vi "conect and open B.vi"(4 "Slot":u32, 5 "Bus":u32, 6 "Remote Machine":string="192.168.1.218", 7 "Card ID":string) -> (0 "error out":errorcluster {"code" format="%.0x"}, 2 "find?":bool, 3 "Output Handle":cluster{"Session":u32, "Card number":u32})   [LabVIEW 2018]
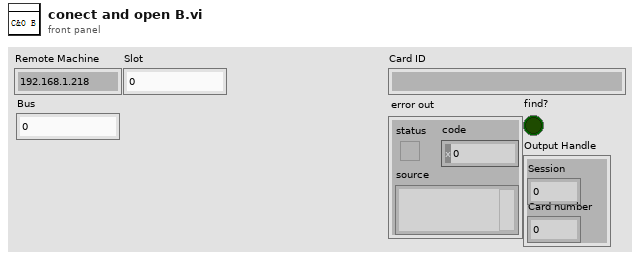
[diagram p1: front panel]
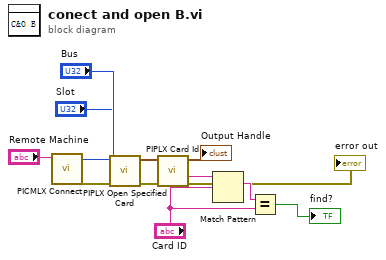
[diagram p0: block diagram]
diagram:
  n1 = call <instrlib>:"PICMLX Connect.vi"("Remote Machine"="Remote Machine") -> ("error out"=w12:errorcluster, "Session"=w13:u32)  [unwired: 8 in]
  n2 = call <instrlib>:"PIPLX Open Specified Card.vi"("error in"=w12, "Slot"="Slot", "Bus"="Bus", "Session"=w13) -> ("error out"=w11:errorcluster, "Output Handle"=w10:cluster{"Session":u32, "Card number":u32})  [unwired: 6 in]
  n3 = call <instrlib>:"PIPLX Card Id.vi"("error in"=w11, "Input Handle"=w10) -> ("error out"=→"error out":errorcluster, "Card ID"=w9:string, "Output Handle"=→"Output Handle":cluster{"Session":u32, "Card number":u32})  [unwired: 7 in]
  n4 = Match Pattern(string=w9, regular expression="Card ID") -> (match substring=w8:string)  [unwired: 1 in, 3 out]
  n5 = Equal?(x=w8, y="Card ID") -> (x = y?=→"find?":bool)
